vi "ConvertTriggerSourceToString.vi"(11 "Trigger Source":T1=enum."Immediate") -> (3 "Trigger Source String":string)   [LabVIEW 2012, in "Keithley-7001.lvlib"]
uses:
  Keithley-7001.lvlib
  Public/Controls/TriggerSource.ctl
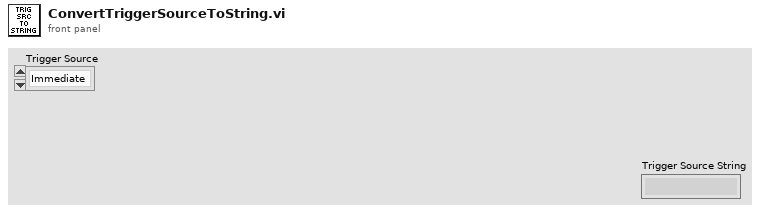
[diagram p1: front panel]
types:
  T1 = typedef "Keithley-7001.lvlib/TriggerSource.ctl" = enum16{"Hold", "Immediate", "Manual", "Bus", "TLink", "External", "Timer"}
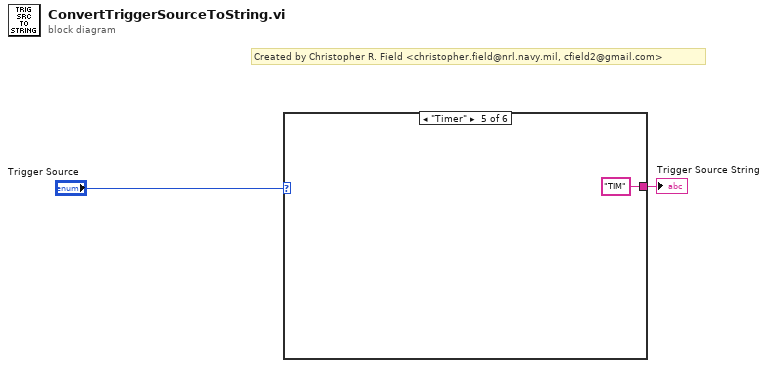
[diagram p0: block diagram]
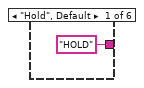
[diagram p2: hidden frame]
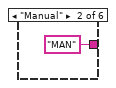
[diagram p3: hidden frame]
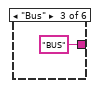
[diagram p4: hidden frame]
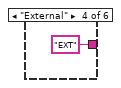
[diagram p5: hidden frame]
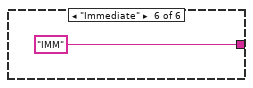
[diagram p6: hidden frame]
diagram:
  # "Created by Christopher R. Field <christopher.field@nrl.navy.mil, cfield2@gmail.com>"
  n1 = case shown="\"Timer\"" "Trigger Source" {
    tunnel: ["HOLD" "MAN" "BUS" "EXT" "TIM" "IMM"] -> w2
    frame "Hold", Default {
    }
    frame "Manual" {
    }
    frame "Bus" {
    }
    frame "External" {
    }
    frame "Timer" {
    }
    frame "Immediate" {
    }
  }
  "Trigger Source String" <- w2
